vi "HFRR ADV v013 new software.vi"() -> ()   [LabVIEW 2025] (continued)
            n3539 = property class="DigNum (strict)"("Numeric Text.Text Colors:Text Color"="NI Text  2") -> ()  [unwired: 2 in, 2 out]
            n3540 = property class="DigNum (strict)"("Numeric Text.Text Colors:Text Color"="NI Text  2") -> ()  [unwired: 2 in, 2 out]
            n3541 = property class="DigNum (strict)"("Numeric Text.Text Colors:Text Color"="NI Text  2") -> ()  [unwired: 2 in, 2 out]
            n3542 = property on="Coefficient Of Friction" class="XYGraph (strict)"("Plot Area:Colors:FG Color"="GFG  2", "Plot Area:Colors:BG Color"="GBG   2") -> ()  [unwired: 2 in, 2 out]
            n3543 = property on="Humidity ( %RH )" class="XYGraph (strict)"("Plot Area:Colors:FG Color"="GFG  2", "Plot Area:Colors:BG Color"="GBG   2") -> ()  [unwired: 2 in, 2 out]
            n3544 = property on="Air Temperature  ( °C )" class="XYGraph (strict)"("Plot Area:Colors:FG Color"="GFG  2", "Plot Area:Colors:BG Color"="GBG   2") -> ()  [unwired: 2 in, 2 out]
            n3545 = property on="Sample Temperature ( °C )" class="XYGraph (strict)"("Plot Area:Colors:FG Color"="GFG  2", "Plot Area:Colors:BG Color"="GBG   2") -> ()  [unwired: 2 in, 2 out]
            n3546 = property class="DigNum (strict)"("Numeric Text.Text Colors:BG Color"="NI BG 2") -> ()  [unwired: 2 in, 2 out]
            n3547 = property class="DigNum (strict)"("Numeric Text.Text Colors:BG Color"="NI BG 2") -> ()  [unwired: 2 in, 2 out]
            n3548 = property class="DigNum (strict)"("Numeric Text.Text Colors:BG Color"="NI BG 2") -> ()  [unwired: 2 in, 2 out]
            n3549 = property class="DigNum (strict)"("Numeric Text.Text Colors:BG Color"="NI BG 2") -> ()  [unwired: 2 in, 2 out]
            n3550 = property class="DigNum (strict)"("Numeric Text.Text Colors:BG Color"="NI BG 2") -> ()  [unwired: 2 in, 2 out]
            n3551 = property class="DigNum (strict)"("Numeric Text.Text Colors:BG Color"="NI BG 2") -> ()  [unwired: 2 in, 2 out]
            n3552 = property class="DigNum (strict)"("Numeric Text.Text Colors:BG Color"="NI BG 2") -> ()  [unwired: 2 in, 2 out]
            n3553 = property class="DigNum (strict)"("Numeric Text.Text Colors:BG Color"="NI BG 2") -> ()  [unwired: 2 in, 2 out]
            n3554 = property class="DigNum (strict)"("Numeric Text.Text Colors:BG Color"="NI BG 2") -> ()  [unwired: 2 in, 2 out]
            n3555 = property class="DigNum (strict)"("Numeric Text.Text Colors:BG Color"="NI BG 2") -> ()  [unwired: 2 in, 2 out]
            n3556 = property class="DigNum (strict)"("Numeric Text.Text Colors:BG Color"="NI BG 2") -> ()  [unwired: 2 in, 2 out]
            n3557 = property class="DigNum (strict)"("Numeric Text.Text Colors:BG Color"="NI BG 2") -> ()  [unwired: 2 in, 2 out]
            n3558 = property class="DigNum (strict)"("Numeric Text.Text Colors:BG Color"="NI BG 2") -> ()  [unwired: 2 in, 2 out]
            n3559 = property class="DigNum (strict)"("Numeric Text.Text Colors:BG Color"="NI BG 2") -> ()  [unwired: 2 in, 2 out]
            n3560 = property class="DigNum (strict)"("Numeric Text.Text Colors:BG Color"="NI BG 2") -> ()  [unwired: 2 in, 2 out]
            n3561 = property class="Bool"("Colors [4]"="Boolean BC T & BG") -> ()  [unwired: 2 in, 2 out]
            n3562 = property on="Save & Continue" class="Bool (strict)"("Colors [4]"="Boolean BC T & BG") -> ()  [unwired: 2 in, 2 out]
            n3563 = property on="Heater Button" class="Bool (strict)"("Colors [4]"="Boolean BC T & BG") -> ()  [unwired: 2 in, 2 out]
            n3564 = property class="Bool"("Colors [4]"="Boolean BC T & BG") -> ()  [unwired: 2 in, 2 out]
            n3565 = property on="Humidity" class="Bool (strict)"("Colors [4]"="Boolean BC T & BG") -> ()  [unwired: 2 in, 2 out]
            n3566 = property class="Bool (strict)"("Colors [4]"="Boolean BC T & BG") -> ()  [unwired: 2 in, 2 out]
            n3567 = property on="RUN" class="Bool (strict)"("Colors [4]"="Boolean BC T & BG") -> ()  [unwired: 2 in, 2 out]
            n3568 = property on="trip1 8" class="Bool (strict)"("Colors [4]"="Boolean BC T & BG") -> ()  [unwired: 2 in, 2 out]
            n3569 = property class="Bool"("Colors [4]"="Boolean BC T & BG") -> ()  [unwired: 2 in, 2 out]
            n3570 = property class="Bool (strict)"("Colors [4]"="Boolean BC T & BG") -> ()  [unwired: 2 in, 2 out]
            n3571 = property on="OPEN 1" class="Bool (strict)"("Colors [4]"="Boolean BC T & BG 2") -> ()  [unwired: 2 in, 2 out]
            n3572 = property on="OPEN 2" class="Bool (strict)"("Colors [4]"="Boolean BC T & BG 2") -> ()  [unwired: 2 in, 2 out]
            n3573 = property on="OPEN 3" class="Bool (strict)"("Colors [4]"="Boolean BC T & BG 2") -> ()  [unwired: 2 in, 2 out]
            n3574 = property on="OPEN 4" class="Bool (strict)"("Colors [4]"="Boolean BC T & BG 2") -> ()  [unwired: 2 in, 2 out]
            n3575 = property on="OPEN" class="Bool (strict)"("Colors [4]"="Boolean BC T & BG 2") -> ()  [unwired: 2 in, 2 out]
            n3576 = property on="rstv2" class="Bool"("Colors [4]"="Boolean BC T & BG 2") -> ()  [unwired: 2 in, 2 out]
            n3577 = property on="RST CP" class="Bool"("Colors [4]"="Boolean BC T & BG 2") -> ()  [unwired: 2 in, 2 out]
            n3578 = property on="RSTV1 3" class="Bool"("Colors [4]"="Boolean BC T & BG 2") -> ()  [unwired: 2 in, 2 out]
            n3579 = property on="RSTV1 2" class="Bool"("Colors [4]"="Boolean BC T & BG 2") -> ()  [unwired: 2 in, 2 out]
          }
          frame #1 {
          }
        }
        n3580 = local read "Quit"() -> (w4456:bool)
      }
    }
    frame Enabled {
    }
  }
  n3581 = while {
    shift-right: [w4474] -> _
    shift-left: _ -> [w4475]
    shift-right: [w4472] -> _
    shift-left: T18 {"Read Heave and Surge"="", "Bytes at Heave Port"=0.0, "Heave and Surge COM Port:"="COM9", "Com Port 2"="COM7", "Residual Due"="", "Heave COM Status 2"=TRUE, "Heave COM Status"=TRUE, "Port 2"=TRUE, "Sway PPR"=6400.0, "Surge PPR"=6400.0, "Heave PPR"=6400.0, "Sway Pitch"=2.0, "Surge Pitch"=3.0, "Heave Pitch"=4.0, "Sway Pulses/mm"=320.0, "Surge Pulses/mm"=1600.0, "Heave Pulses/mm"=1600.0, "inner loop"=0.0, "Read Heave and Surge 2"="", "String 36"="", "Write S"=FALSE, "WriteCC1"=[""], "Heave COM Loop"=0, "LastCom"="", "EXIT"=FALSE, "Error Heave"={"status"=TRUE, "code"=-1073807343, "source"=""}} -> [w4471]
    shift-right: [w4469] -> _
    shift-left: enum16{"init", "MAIN", "Panel Close"}."init" -> [w4470]
    stop <- w4473 stop-if-true
    n3582 = case shown="\"MAIN\"" w4470 {
      tunnel: w4475 -> [w4489 w4504 w4565 w4567]
      tunnel: [w4483 w4513 w4565 w4567] -> w4474
      tunnel: [_ _ TRUE _] -> w4473
      tunnel: [w4479 w4510 w4563 w4566] -> w4472
      tunnel: w4471 -> [w4486 w4503 w4563 w4566]
      tunnel: [enum16{"init", "MAIN", "Panel Close"}."MAIN" w4497 _ _] -> w4469
      frame "init" {
        n3583 = Bundle By Name(cluster=w4486, "Heave and Surge COM Port:"="C3 :") -> (w4485:T18)
        n3584 = call "Instrument fgv.vi"("Enum"=T30."INIT", "error in (no error) 2"=w4489, "INPUT"=w4485) -> ("error"=w4487:errorcluster, "output"=w4482:T18)  [unwired: 6 in, 1 out]
        n3585 = case shown="Error" w4487 {
          selector: w4487 -> [w4491 _]
          tunnel: [w4491 w4495] -> w4483
          tunnel: w4482 -> [w4490 w4493]
          tunnel: [w4490 w4492] -> w4480
          frame No Error {
          }
          frame Error {
            n3586 = call "Instrument fgv.vi"("Enum"=T30."ERROR INIT", "INPUT"=w4493) -> ("error"=w4496:errorcluster, "output"=w4492:T18)  [unwired: 7 in, 1 out]
            n3587 = call <vilib>:"Clear Errors.vi"("error in (no error)"=w4496) -> ("error out"=w4495:errorcluster)  [unwired: 5 in, 1 out]
          }
        }
        n3588 = local read "LastCom"() -> (w4478:string)
        n3589 = Unbundle By Name(w4480) -> ("Heave COM Status 2"=→"COM Status" →"Instrument Status":bool, "Error Heave"=→"Error":errorcluster)  [unwired: 1 out]
        n3590 = Bundle By Name(cluster=w4480, "LastCom"=w4478) -> (w4479:T18)
      }
      frame "MAIN" {
        n3591 = Unbundle By Name(w4503) -> ("Com Port 2"=w4515:refnum<visa-resource-name>)
        n3592 = local write "Com Port 4"(w4515) -> ()
        n3593 = local read "C3 :"() -> (w4501:refnum<visa-resource-name>)
        n3594 = Bundle By Name(cluster=w4503, "Heave and Surge COM Port:"=w4501) -> (w4502:T18)
        n3595 = Equal?(x=w4515, y=w4501) -> (x = y?=w4514:bool)
        n3596 = case shown="True" w4514 {
          tunnel: [w4519 w4536] -> w4513
          tunnel: w4504 -> [w4520 w4542]
          tunnel: w4502 -> [w4518 w4540]
          tunnel: [w4517 w4535] -> w4510
          frame False {
            n3597 = call <vilib>:"Clear Errors.vi"("error in (no error)"=w4520) -> ("error out"=w4516:errorcluster)  [unwired: 5 in, 1 out]
            n3598 = call "Instrument fgv.vi"("Enum"=T30."ERROR INIT", "error in (no error) 2"=w4516, "INPUT"=w4518) -> ("error"=w4522:errorcluster, "output"=w4517:T18)  [unwired: 6 in, 1 out]
            n3599 = call <vilib>:"Clear Errors.vi"("error in (no error)"=w4522) -> ("error out"=w4519:errorcluster)  [unwired: 5 in, 1 out]
          }
          frame True {
            n3600 = call "Instrument fgv.vi"("Enum"=T30."READ", "error in (no error) 2"=w4542, "INPUT"=w4540) -> ("error"=w4541:errorcluster, "output"=w4532:T18)  [unwired: 6 in, 1 out]
            n3601 = Bundle By Name(cluster=w4532, "String 36"="String 11") -> (w4531:T18)
            n3602 = case shown="True" "Write S" {
              selector: "Write S" -> [_ w4562]
              tunnel: w4541 -> [w4555 w4561]
              tunnel: [w4555 w4560] -> w4528
              tunnel: w4531 -> [w4554 w4557]
              tunnel: [w4554 w4556] -> w4527
              frame False {
              }
              frame True {
                n3603 = Not(x=w4562) -> (.not. x?=w4558:bool)
                n3604 = local write "Write S"(w4558) -> ()
                n3605 = call "Instrument fgv.vi"("Enum"=T30."MANUAL WRITE", "error in (no error) 2"=w4561, "INPUT"=w4557) -> ("error"=w4560:errorcluster, "output"=w4556:T18)  [unwired: 6 in, 1 out]
              }
            }
            n3606 = Array Size(array="WriteHumidity") -> (size(s)=w4525:i32)
            n3607 = Greater Than 0?(x=w4525) -> (x > 0?=w4523:bool)
            n3608 = call "Instrument fgv.vi"("Enum"=T30."WRITE", "error in (no error) 2"=w4528, "WriteCC1"="WriteHumidity", "INPUT"=w4527) -> ("error"=w4538:errorcluster, "WriteCC1 2"=w4526:string[], "output"=w4537:T18)  [unwired: 5 in]
            n3609 = case shown="True" w4523 {
              tunnel: w4526 -> [_ w4544]
              frame False {
              }
              frame True {
                n3610 = local write "WriteHumidity"(w4544) -> ()
              }
            }
            n3611 = case shown="Error" w4538 {
              selector: w4538 -> [w4545 w4548]
              tunnel: w4537 -> [w4546 w4553]
              tunnel: [w4546 w4552] -> w4535
              tunnel: [w4545 w4550] -> w4536
              frame No Error {
              }
              frame Error {
                n3612 = call <vilib>:"Clear Errors.vi"("error in (no error)"=w4548) -> ("error out"=w4547:errorcluster)  [unwired: 5 in, 1 out]
                n3613 = call "Instrument fgv.vi"("Enum"=T30."ERROR INIT", "error in (no error) 2"=w4547, "INPUT"=w4553) -> ("error"=w4551:errorcluster, "output"=w4552:T18)  [unwired: 6 in, 1 out]
                n3614 = call <vilib>:"Clear Errors.vi"("error in (no error)"=w4551) -> ("error out"=w4550:errorcluster)  [unwired: 5 in, 1 out]
              }
            }
            n3615 = Unbundle By Name(w4535) -> ("LastCom"=→"LastCom":string, "Read Heave and Surge"=→"Read Humidity":string)
          }
        }
        n3616 = Unbundle By Name(w4510) -> ("Heave COM Status 2"=w4512:bool, "Heave COM Status"=w4511:bool, "Error Heave"=w4508:errorcluster, "Bytes at Heave Port"=→"Bytes at Humidity Port":dbl)
        n3617 = Unbundle By Name(w4508) -> ("status"=→"Humidity Port":bool)
        n3618 = Not(x=w4511) -> (.not. x?=w4505:bool)
        n3619 = local write "Error"(w4508) -> ()
        n3620 = Not(x=w4512) -> (.not. x?=w4506:bool)
        n3621 = local write "Instrument Status"(w4505) -> ()
        n3622 = local write "COM Status"(w4506) -> ()
        n3623 = local read "Quit"() -> (w4498:bool)
        n3624 = Select(t=enum16{"init", "MAIN", "Panel Close"}."Panel Close", s=w4498, f=enum16{"init", "MAIN", "Panel Close"}."MAIN") -> (s? t:f=w4497:enum16{"init", "MAIN", "Panel Close"})
      }
      frame "Panel Close" {
      }
      frame Default {
      }
    }
  }
  n3625 = while {
    stop <- w4593 stop-if-true
    n3626 = local read "Read Humidity"() -> (w4574:string)
    n3627 = call <vilib>:"High Resolution Polling Wait.vi"("seconds to wait"=0.1) -> ()  [unwired: 10 in, 1 out]
    n3628 = Spreadsheet String To Array(delimiter (Tab)=",", format string="", spreadsheet string=w4574, array type (2D Dbl)=string[] []) -> (array=w4588:string[])
    n3629 = for {
      tunnel: w4588 -> [w4598] mode=indexing
      tunnel: string[] ["STATE;", "SET;", "RH;", "T;", "AMB_RH;", "AMB_T;", "PUMP;", "FAN_IN;", "FAN_OUT;", "DEHUM;", "CURRENT;", "STALL;"] -> [w4597] mode=indexing
      tunnel: [w4596] -> w4587 mode=indexing
      n3630 = Match Pattern(string=w4598, regular expression=w4597) -> (after substring=w4596:string)  [unwired: 1 in, 3 out]
    }
    n3631 = Index Array(array=w4587) -> (element #1=→"STATE :":string, element #2=→"SET :":string, element #3=w4576:string, element #4=→"T :":string, element #5=w4573:string, element #6=→"AMB_T :":string, element #7=→"PUMP :":string, element #8=→"FAN_IN :":string, element #9=→"FAN_OUT :":string, element #10=→"DEHUM :":string, element #11=→"CURRENT :":string, element #12=→"STALL :":string)  [unwired: 12 in]
    "RH :" <- w4576
    "AMB_RH :" <- w4573
    n3632 = Fract/Exp String To Number(string=w4576) -> (number=w4568:dbl)  [unwired: 3 in, 1 out]
    n3633 = Fract/Exp String To Number(string=w4573) -> (number=w4572:dbl)  [unwired: 3 in, 1 out]
    n3634 = local write "Ambient Humidity :"(w4572) -> ()
    n3635 = Equal?(x=w4568, y=0.0) -> (x = y?=w4570:bool)
    n3636 = case shown="True" w4570 {
      tunnel: [w4594 w4595] -> w4569
      tunnel: w4568 -> [w4594 _]
      frame False {
        (unwired) 0.0
        "Humidity temp" <- w4594
      }
      frame True {
        n3637 = local read "Humidity temp"() -> (w4595:dbl)
      }
    }
    "RH Numeric:" <- w4569
    n3638 = local read "Quit"() -> (w4593:bool)
  }
  n3639 = disable-structure shown="Disabled" {
    frame Disabled {
      n3640 = while {
        tunnel: [w4832] -> _
        i -> [w4832]
        stop <- w4829 stop-if-true
        n3641 = local read "powstat"() -> (w4830:bool)
        n3642 = case shown="True" w4830 {
          frame False {
          }
          frame True {
            n3643 = local read "RUN"() -> (w4833:bool)
            n3644 = case shown="True" w4833 {
              frame False {
                w4863 = 65.0 ("y")
                n3645 = local read "Set Hz"() -> (w4891:dbl)
                n3646 = local read "NORMAL LOAD"() -> (w4892:dbl)
                n3647 = Multiply(x=w4891, y=60.0) -> (x*y=w4898:dbl)
                n3648 = Multiply(x=1.2 ("y"), y=0.949) -> (x*y=w4867:dbl)
                n3649 = Multiply(x=1.2 ("y"), y=0.8166) -> (x*y=w4871:dbl)
                n3650 = Multiply(x=1.2 ("y"), y=0.851) -> (x*y=w4866:dbl)
                n3651 = local read "FF 2"() -> (w4890:dbl)
                n3652 = Absolute Value(x=w4898) -> (abs(x)=w4896:dbl)
                n3653 = case shown="13.." w4890 {
                  tunnel: [1 2 3] -> w4888
                  frame 0..10, Default {
                    # "Normal"
                  }
                  frame 11, 12 {
                  }
                  frame 13.. {
                  }
                }
                "FF STATE" <- w4888
                n3654 = local read "TEMP"() -> (w4851:dbl)
                n3655 = local read item#-1() -> (w4865)
                n3656 = Less?(x=w4865, y=w4871) -> (x < y?=w4868:bool)
                n3657 = In Range and Coerce(upper limit=w4867, x=w4865, lower limit=w4866) -> (In Range?=w4869:bool)  [unwired: 1 out]
                n3658 = case shown="3601.." w4896 {
                  tunnel: [1 2 3] -> w4894
                  frame 0..3000, Default {
                    # "Normal"
                  }
                  frame 3001..3600 {
                  }
                  frame 3601.. {
                  }
                }
                n3659 = case shown="11.." w4892 {
                  tunnel: [1 3] -> w4893
                  frame 1..10, Default {
                  }
                  frame 11.. {
                  }
                }
                "NL STATE" <- w4893
                n3660 = Multiply(x=1.2 ("y"), y=0.95) -> (x*y=w4881:dbl)
                n3661 = Multiply(x=w4863, y=0.954) -> (x*y=w4855:dbl)
                n3662 = Or(x=w4868, y=w4869) -> (x .or. y?=w4870:bool)
                n3663 = Greater Or Equal?(x=w4865, y=w4881) -> (x >= y?=w4878:bool)
                n3664 = Multiply(x=w4863, y=0.99) -> (x*y=w4852:dbl)
                n3665 = Greater Or Equal?(x=w4851, y=w4852) -> (x >= y?=w4857:bool)
                n3666 = Greater Or Equal?(x=w4851, y=w4855) -> (x >= y?=w4854:bool)
                n3667 = case shown="0, 1, Default" w4865 {
                  tunnel: [1 3] -> w4882
                  frame 0, 1, Default {
                  }
                  frame 2.. {
                  }
                }
                n3668 = case shown="True" w4878 {
                  tunnel: [1 3] -> w4883
                  frame False {
                  }
                  frame True {
                  }
                }
                n3669 = case shown="True" w4870 {
                  tunnel: [1 2] -> w4884
                  frame False {
                  }
                  frame True {
                  }
                }
                n3670 = case shown="..0" w4851 {
                  tunnel: [2 3 3 1] -> w4858
                  frame 61, 62 {
                  }
                  frame 63.. {
                  }
                  frame ..0 {
                  }
                  frame 10..60, Default {
                  }
                }
                n3671 = case shown="True" w4857 {
                  tunnel: [1 3] -> w4859
                  frame False {
                  }
                  frame True {
                  }
                }
                n3672 = Number To Decimal String(number=w4894) -> (decimal integer string=w4895:string)  [unwired: 1 in]
                n3673 = case shown="True" w4854 {
                  tunnel: [1 2] -> w4860
                  frame False {
                  }
                  frame True {
                  }
                }
                n3674 = Number To Decimal String(number=1) -> (decimal integer string=→"Air temp":string)  [unwired: 1 in]
                n3675 = Number To Decimal String(number=w4888) -> (decimal integer string=→"ff_st":string)  [unwired: 1 in]
                n3676 = local write "sp_st"(w4895) -> ()
                n3677 = Number To Decimal String(number=w4893) -> (decimal integer string=→"nl_st":string)  [unwired: 1 in]
                n3678 = Build Array(w4858, w4859, w4860) -> (w4861:i32[])
                n3679 = Build Array(w4882, w4883, w4884) -> (w4885:i32[])
                n3680 = Array Max & Min(array=w4861) -> (max value=w4862:i32)  [unwired: 3 out]
                n3681 = Array Max & Min(array=w4885) -> (max value=w4886:i32)  [unwired: 3 out]
                n3682 = Number To Decimal String(number=w4862) -> (decimal integer string=w4850:string)  [unwired: 1 in]
                n3683 = Number To Decimal String(number=w4886) -> (decimal integer string=→"Stroke Ln 2":string)  [unwired: 1 in]
                n3684 = local write "temp_st"(w4850) -> ()
              }
              frame True {
                w4948 = 65.0 ("y")
                # "Healthy -1\nWarning -2\nError -3"
                n3685 = local read "TEMP"() -> (w4959:dbl)
                n3686 = local read "NORMAL LOAD"() -> (w4963:dbl)
                n3687 = local read "Set Hz"() -> (w4961:dbl)
                n3688 = Multiply(x=1.2 ("y"), y=0.949) -> (x*y=w4943:dbl)
                n3689 = Multiply(x=1.2 ("y"), y=0.8166) -> (x*y=w4939:dbl)
                n3690 = Multiply(x=1.2 ("y"), y=0.851) -> (x*y=w4944:dbl)
                n3691 = Multiply(x=w4948, y=0.954) -> (x*y=w4955:dbl)
                n3692 = Multiply(x=w4948, y=0.99) -> (x*y=w4958:dbl)
                n3693 = Greater Or Equal?(x=w4959, y=w4958) -> (x >= y?=w4953:bool)
                n3694 = Multiply(x=w4961, y=60.0) -> (x*y=w4967:dbl)
                n3695 = Greater Or Equal?(x=w4959, y=w4955) -> (x >= y?=w4956:bool)
                n3696 = local read "FF 2"() -> (w4962:dbl)
                n3697 = local read item#-1() -> (w4945)
                n3698 = Less?(x=w4945, y=w4939) -> (x < y?=w4942:bool)
                n3699 = In Range and Coerce(upper limit=w4943, x=w4945, lower limit=w4944) -> (In Range?=w4941:bool)  [unwired: 1 out]
                n3700 = Absolute Value(x=w4967) -> (abs(x)=w4965:dbl)
                n3701 = case shown="63.." w4959 {
                  tunnel: [2 3 3 1] -> w4952
                  frame 61, 62 {
                  }
                  frame 63.. {
                  }
                  frame ..0 {
                  }
                  frame 10..60, Default {
                  }
                }
                n3702 = case shown="True" w4953 {
                  tunnel: [1 3] -> w4951
                  frame False {
                  }
                  frame True {
                  }
                }
                n3703 = case shown="True" w4956 {
                  tunnel: [1 2] -> w4950
                  frame False {
                  }
                  frame True {
                  }
                }
                n3704 = Multiply(x=1.2 ("y"), y=0.95) -> (x*y=w4929:dbl)
                n3705 = case shown="1..10, Default" w4963 {
                  tunnel: [1 3] -> w4970
                  frame 1..10, Default {
                  }
                  frame 11.. {
                  }
                }
                n3706 = case shown="0..10, Default" w4962 {
                  tunnel: [1 2 3] -> w4969
                  frame 0..10, Default {
                  }
                  frame 11, 12 {
                  }
                  frame 13.. {
                  }
                }
                n3707 = case shown="3601.." w4965 {
                  tunnel: [1 2 3] -> w4964
                  frame 0..3000, Default {
                    # "Normal"
                  }
                  frame 3001..3600 {
                  }
                  frame 3601.. {
                  }
                }
                n3708 = Or(x=w4942, y=w4941) -> (x .or. y?=w4940:bool)
                n3709 = Greater Or Equal?(x=w4945, y=w4929) -> (x >= y?=w4932:bool)
                n3710 = case shown="0, 1, Default" w4945 {
                  tunnel: [1 3] -> w4928
                  frame 0, 1, Default {
                  }
                  frame 2.. {
                  }
                }
                n3711 = case shown="True" w4932 {
                  tunnel: [1 3] -> w4927
                  frame False {
                  }
                  frame True {
                  }
                }
                n3712 = case shown="True" w4940 {
                  tunnel: [1 2] -> w4926
                  frame False {
                  }
                  frame True {
                  }
                }
                n3713 = Build Array(w4952, w4951, w4950) -> (w4949:i32[])
                n3714 = Number To Decimal String(number=w4964) -> (decimal integer string=→"sp_st":string)  [unwired: 1 in]
                n3715 = Array Max & Min(array=w4949) -> (max value=w4946:i32)  [unwired: 3 out]
                "TEMP STATE" <- w4946
                n3716 = Number To Decimal String(number=w4970) -> (decimal integer string=w4973:string)  [unwired: 1 in]
                n3717 = Number To Decimal String(number=w4969) -> (decimal integer string=w4971:string)  [unwired: 1 in]
                n3718 = Number To Decimal String(number=w4946) -> (decimal integer string=→"temp_st":string)  [unwired: 1 in]
                n3719 = Build Array(w4928, w4927, w4926) -> (w4925:i32[])
                n3720 = local write "nl_st"(w4973) -> ()
                n3721 = local write "ff_st"(w4971) -> ()
                n3722 = Number To Decimal String(number=1) -> (decimal integer string=w4968:string)  [unwired: 1 in]
                n3723 = Array Max & Min(array=w4925) -> (max value=w4924:i32)  [unwired: 3 out]
                n3724 = local write "Air temp"(w4968) -> ()
                n3725 = Number To Decimal String(number=w4924) -> (decimal integer string=w4923:string)  [unwired: 1 in]
                n3726 = local write "Stroke Ln 2"(w4923) -> ()
              }
            }
            n3727 = local read "Stroke Ln 2"() -> (w4835:string)
            n3728 = local read "nl_st"() -> (w4841:string)
            n3729 = local read "ff_st"() -> (w4838:string)
            n3730 = local read "sp_st"() -> (w4839:string)
            n3731 = local read "temp_st"() -> (w4840:string)
            n3732 = local read "Air temp"() -> (w4834:string)
            n3733 = Replace Array Subset(array="in", new element #1=w4841, index #1=1 ("index"), new element #2=w4838, index #2=2 ("index"), new element #3=w4840, index #3=3 ("index"), new element #4=w4839, index #4=4 ("index"), new element #5=w4835, index #5=5 ("index"), new element #6=w4834, index #6=6 ("index"), new element #7="Sensor State" ("new element/subarray"), index #7=0 ("index")) -> (→"out":string[])
          }
        }
        n3734 = Wait (ms)(milliseconds to wait=u32 10) -> ()  [unwired: 1 out]
        n3735 = local read "Quit"() -> (w4829:bool)
      }
      n3736 = while {
        stop <- w4804 stop-if-true
        n3737 = local read "run replace"() -> (w4806:bool)
        n3738 = Wait (ms)(milliseconds to wait=u32 100) -> ()  [unwired: 1 out]
        n3739 = Equal?(x="FLAG 2", y=0.0) -> (x = y?=w4807:bool)
        n3740 = case shown="True" w4807 {
          frame False {
          }
          frame True {
            n3741 = local write "FLAG 2"(100.0 ("FLAG 2")) -> ()
            n3742 = call <vilib>:"Read Characters From File.vi"("file path (dialog if empty)"=path "C:/LAB-IQ-NXT/WO 2449 TT.sig", "convert eol? (no:F)"=FALSE ("append to file? (new file:F)")) -> ("character string"=w4810:string)  [unwired: 4 in, 3 out]
            n3743 = call <vilib>:"Read Characters From File.vi"("file path (dialog if empty)"=path "C:/LAB-IQ-NXT/WO 2449 TRH.sig", "convert eol? (no:F)"=FALSE ("append to file? (new file:F)")) -> ("character string"=w4811:string)  [unwired: 4 in, 3 out]
            n3744 = Decimal String To Number(string=w4810) -> (number=w4812:i32)  [unwired: 2 in, 1 out]
            n3745 = local write "Total No. of Tests"(w4812) -> ()
            n3746 = Decimal String To Number(string=w4811) -> (number=w4815:i32)  [unwired: 2 in, 1 out]
            n3747 = local write "SEN.RUN HRS"(w4815) -> ()
          }
        }
        n3748 = case shown="True" w4806 {
          frame False {
          }
          frame True {
            n3749 = Equal?(x="FLAG 4", y=0.0) -> (x = y?=w4819:bool)
            n3750 = case shown="False" w4819 {
              frame False {
                n3751 = Get Date/Time In Seconds() -> (seconds since 1Jan1904=w4825:timestamp)
                n3752 = local read "START 3"() -> (w4823:dbl)
                n3753 = To Double Precision Float(number=w4825) -> (double precision float=w4824:dbl)
                n3754 = Subtract(x=w4824, y=w4823) -> (x-y=→"SENSOR TIME":dbl)
              }
              frame True {
                n3755 = Get Date/Time In Seconds() -> (seconds since 1Jan1904=w4827:timestamp)
                n3756 = local write "FLAG 4"(100.0 ("FLAG")) -> ()
                n3757 = To Double Precision Float(number=w4827) -> (double precision float=→"START 3":dbl)
              }
            }
          }
        }
        n3758 = local read "Quit"() -> (w4804:bool)
      }
      n3759 = while {
        shift-right: [w4604] -> _
        shift-left: _ -> [w4605]
        tunnel: [w4600] -> _
        i -> [w4600]
        stop <- w4599 stop-if-true
        n3760 = Wait (ms)(milliseconds to wait=u32 50 ("Refresh Rate (ms)")) -> ()  [unwired: 1 out]
        n3761 = local read "Json End Flg"() -> (w4601:bool)
        n3762 = Not(x="Upld AR 2") -> ()  [unwired: 1 out]
        n3763 = local read "Upld AR 2"() -> (w4602:bool)
        n3764 = call "Elapsed Time9"("Time Target (s)"="Sen.Upload Rate (s)", "Reset"=FALSE, "Auto Reset"=TRUE) -> ("Time has Elapsed"=w4611:bool)  [unwired: 9 in, 7 out]
        n3765 = Or(x=w4611, y=w4601) -> (x .or. y?=w4607:bool)
        n3766 = case shown="True" w4607 {
          frame False {
          }
          frame True {
            w4703 = "\"SensorName\":\"" ("string")
            w4673 = " \"},{"
            w4698 = "\",\"SensorState\":\""
            w4700 = "\",\"SensorModelNumber\":\"" ("string")
            w4699 = "\",\"SensorRuntimeHours\":\"" ("string")
            n3767 = local read "model num"() -> (w4697:string[])
            n3768 = local read "Sensor name"() -> (w4716:string[])
            n3769 = local read "run"() -> (w4687:string[])
            n3770 = local read "SENSOR TIME"() -> (w4643:dbl)
            n3771 = local read "out"() -> (w4636:string[])
            n3772 = local read "Total No. of Tests"() -> (w4641:dbl)
            n3773 = Select(t=60.0, s="Run test 3", f=3600.0) -> (s? t:f=w4651:dbl)
            n3774 = Index Array(array=w4697, index #1=1 ("index")) -> (element #1=w4696:string, element #2=w4695:string, element #3=w4694:string, element #4=w4693:string, element #5=w4692:string, element #6=w4691:string)  [unwired: 5 in]
            n3775 = Index Array(array=w4687, index #1=1 ("index")) -> (element #1=w4686:string, element #2=w4685:string, element #3=w4684:string, element #4=w4683:string, element #5=w4682:string, element #6=w4681:string)  [unwired: 5 in]
            n3776 = Index Array(array=w4716, index #1=1 ("index")) -> (element #1=w4715:string, element #2=w4714:string, element #3=w4713:string, element #4=w4712:string, element #5=w4702:string, element #6=w4701:string)  [unwired: 5 in]
            n3777 = Index Array(array=w4636, index #1=1 ("index")) -> (element #1=w4668:string, element #2=w4667:string, element #3=w4666:string, element #4=w4665:string, element #5=w4664:string, element #6=w4663:string)  [unwired: 5 in]
            n3778 = local read "SEN.RUN HRS"() -> (w4639:dbl)
            n3779 = Divide(x=w4643, y=w4651) -> (x/y=w4650:dbl)
            n3780 = Increment(x=w4650) -> (x+1=w4646:dbl)
            n3781 = Number To Decimal String(number=w4646) -> (decimal integer string=→"run hrs":string)  [unwired: 1 in]
            n3782 = Divide(x=w4639, y=3600.0 ("f")) -> (x/y=w4634:dbl)
            n3783 = Round To Nearest(number=w4634) -> (nearest integer value=w4632:dbl)
            n3784 = Number To Decimal String(number=w4632) -> (decimal integer string=w4633:string)  [unwired: 1 in]
            n3785 = Number To Decimal String(number=w4641) -> (decimal integer string=w4642:string)  [unwired: 1 in]
            n3786 = local read "Model No"() -> (w4647:string)
            n3787 = local read "UUID"() -> (w4742:string)
            n3788 = local read "Serial No"() -> (w4746:string)
            n3789 = local read "Secret Key"() -> (w4747:string)
            n3790 = Concatenate Strings("\",\"MachineSerialNumber\":\"" ("string"), w4746) -> (w4750:string)
            n3791 = Concatenate Strings("\",\"ModelNumber\":\"" ("string"), w4647) -> (w4648:string)
            n3792 = Concatenate Strings("\",\"MachineRuntimeHours\":\"" ("string"), w4633) -> (w4751:string)
            n3793 = Concatenate Strings("\",\"MachineRuntimeCycles\":\"", w4642) -> (w4744:string)
            n3794 = Concatenate Strings(w4700, w4696) -> (w4730:string)
            n3795 = Concatenate Strings(w4699, w4686) -> (w4731:string)
            n3796 = Concatenate Strings(w4698, w4668) -> (w4729:string)
            n3797 = Concatenate Strings(w4750, w4648, w4751, w4744) -> (w4753:string)
            n3798 = Concatenate Strings(w4700, w4695) -> (w4727:string)
            n3799 = Concatenate Strings(w4699, w4685) -> (w4726:string)
            n3800 = Concatenate Strings(w4698, w4667) -> (w4728:string)
            n3801 = Concatenate Strings(w4700, w4694) -> (w4722:string)
            n3802 = Concatenate Strings(w4699, w4684) -> (w4723:string)
            n3803 = Concatenate Strings(w4698, w4666) -> (w4721:string)
            n3804 = Concatenate Strings(w4700, w4693) -> (w4719:string)
            n3805 = Concatenate Strings(w4699, w4683) -> (w4718:string)
            n3806 = Concatenate Strings(w4698, w4665) -> (w4720:string)
            n3807 = Concatenate Strings(w4730, w4731, w4729) -> (w4732:string)
            n3808 = Concatenate Strings(w4700, w4692) -> (w4709:string)
            n3809 = Concatenate Strings(w4699, w4682) -> (w4710:string)
            n3810 = Concatenate Strings(w4700, w4691) -> (w4706:string)
            n3811 = Concatenate Strings(w4699, w4681) -> (w4705:string)
            n3812 = Concatenate Strings(w4698, w4664) -> (w4708:string)
            n3813 = Concatenate Strings(w4698, w4663) -> (w4707:string)
            n3814 = Concatenate Strings("{\"SecretKey\":\"", w4747, w4753, "\",\"UUID\" : \"", w4742, "\",\"SensorInformation\":", "[{" ("string")) -> (w4680:string)
            n3815 = Concatenate Strings(w4727, w4726, w4728) -> (w4725:string)
            n3816 = Concatenate Strings(w4722, w4723, w4721) -> (w4724:string)
            n3817 = Concatenate Strings(w4719, w4718, w4720) -> (w4717:string)
            n3818 = Concatenate Strings(w4709, w4710, w4708) -> (w4711:string)
            n3819 = Concatenate Strings(w4706, w4705, w4707) -> (w4704:string)
            n3820 = Concatenate Strings(w4703, w4715, w4732, w4673) -> (w4679:string)
            n3821 = Concatenate Strings(w4703, w4714, w4725, w4673) -> (w4678:string)
            n3822 = Concatenate Strings(w4703, w4713, w4724, w4673) -> (w4677:string)
            n3823 = Concatenate Strings(w4703, w4712, w4717, w4673) -> (w4676:string)
            n3824 = Concatenate Strings(w4703, w4702, w4711, w4673) -> (w4675:string)
            n3825 = Concatenate Strings(w4703, w4701, w4704, "\"}" ("string")) -> (w4674:string)
            n3826 = Concatenate Strings(w4680, w4679, w4678, w4677, w4676, w4675, w4674, "]}" ("string")) -> (w4671:string)
            n3827 = local read "SEN.RUN HRS"() -> (w4638:dbl)
            n3828 = disable-structure shown="Disabled" {
              frame Disabled {
                n3829 = local read "state"() -> (w4757:string[])
                n3830 = Delete From Array(array=w4757, index=0) -> (array with subset deleted=w4755:string[])  [unwired: 1 in, 1 out]
                n3831 = for {
                  N: 6 -> [_]
                  tunnel: w4755 -> [w4768] mode=indexing
                  tunnel: [w4767] -> w4754 mode=indexing
                  n3832 = Equal?(x=w4768, y="Warning") -> (x = y?=w4764:bool)
                  n3833 = Equal?(x=w4768, y="Healthy") -> (x = y?=w4761:bool)
                  n3834 = Select(t="2" ("y"), s=w4764, f="3" ("y")) -> (s? t:f=w4759:string)
                  n3835 = Select(t="1" ("y"), s=w4761, f=w4759) -> (s? t:f=w4767:string)
                }
                "state1" <- w4754
              }
              frame Enabled {
              }
            }
            n3836 = stacked-sequence {
              tunnel: w4671 -> [w4779 _ _]
              tunnel: [_ _ w4795] -> _
              frame #0 {
                (unwired) FALSE ("convert eol (F)")
                w4781 = enum16{"start", "end", "current"}."start" ("pos mode (0:2)")
                n3837 = local read "Path"() -> (w4775:path)
                n3838 = Path To String(path=w4775) -> (string=w4787:string)
                n3839 = Concatenate Strings(w4787, "\\", "Sensor File Name") -> (w4788:string)
                n3840 = local write "standard output 2"(" ") -> ()
                n3841 = String To Path(string=w4788) -> (path=w4778:path)
                n3842 = call <vilib>:"Open_Create_Replace File.vi"("advisory dialog? (display:T)"=FALSE, "function (open:0)"=T31."create or replace", "file path"=w4778) -> ("error out"=w4791:errorcluster, "refnum"=w4790:refnum<file>)  [unwired: 5 in, 2 out]
                n3843 = Set File Position(refnum=w4790, from (0:start)=w4781, error in=w4791) -> (refnum out=w4771:refnum<file>, error out=w4770:errorcluster)  [unwired: 1 in]
                n3844 = Write to Binary File(file (use dialog)=w4771, data=" ", error in=w4770, 5:FALSE ("prepend array or string size? (T)")) -> (refnum out=w4782:refnum<file>, error out=w4783:errorcluster)  [unwired: 2 in, 1 out]
                n3845 = Set File Position(offset (in bytes) (0)=w4781, refnum=w4782, error in=w4783) -> (refnum out=w4774:refnum<file>, error out=w4773:errorcluster)  [unwired: 1 in]
                n3846 = Write to Binary File(file (use dialog)=w4774, data=w4779, error in=w4773, 5:FALSE ("prepend array or string size? (T)")) -> (error out=w4777:errorcluster)  [unwired: 2 in, 2 out]
                n3847 = flat-sequence {
                  tunnel: w4778 -> [w4793]
                  tunnel: w4777 -> [_]
                  frame #0 {
                    n3848 = call <vilib>:"Read Characters From File.vi"("file path (dialog if empty)"=w4793) -> ("character string"=→"Sensor Health JSON string":string)  [unwired: 5 in, 3 out]
                  }
                }
                "SinglePoint  2" <- w4779
              }
              frame #1 {
              }
              frame #2 {
                (unwired) "\"Stored\": true" ("string")
                n3849 = call <vilib>:"System Exec.vi"("run minimized? (F)"=TRUE, "wait until completion? (T)"=TRUE, "working directory"=path "C:/LAB-IQ-NXT", "command line"="C:\\LAB-IQ-NXT\\JPostH.bat") -> ("standard error"=→"Respose From Server 2":string, "standard output"=w4798:string)  [unwired: 4 in, 2 out]
                "standard output 2" <- w4798
                n3850 = Match Pattern(string=w4798, regular expression="JSONH Check String") -> (match substring=w4796:string, offset past match=w4795:i32)  [unwired: 1 in, 2 out]
                n3851 = Equal?(x=w4796, y="JSONH Check String") -> (x = y?=→"Upload \nConfirmed 2":bool)
              }
            }
            n3852 = Divide(x=w4638, y=3600.0 ("f")) -> (x/y=w4631:dbl)
            n3853 = local read "run time"() -> (w4688:string[])
            n3854 = Round To Nearest(number=w4631) -> (nearest integer value=w4630:dbl)
            n3855 = Number To Decimal String(number=w4630) -> (decimal integer string=w4629:string)  [unwired: 1 in]
            n3856 = Index Array(array="Sensor Information", index (col) #1=0 ("disabled index (col)"), index (col) #2=1 ("index (col)"), index (col) #3=2 ("index (col)"), index (col) #4=3 ("index (col)")) -> (element #1=→"Sensor name":string[], element #2=→"model num":string[], element #3=→"run time":string[], element #4=→"state":string[])  [unwired: 4 in]
            n3857 = Insert Into Array(array=w4688, index=1, new element #1=w4629, new element #2=w4629, new element #3=w4629, new element #4=w4629, new element #5=w4629, new element #6=w4629) -> (w4653:string[])
            "run" <- w4653
            n3858 = local read "out"() -> (w4635:string[])
            n3859 = local read "Sensor Information"() -> (w4655:string[][])
            n3860 = Replace Array Subset(array=w4655, new element #1=w4653, index (col) #1=2 ("disabled index (col)"), new element #2=w4635, index (col) #2=3 ("index (col)")) -> (w4654:string[][])  [unwired: 2 in]
            n3861 = local write "Sensor Information"(w4654) -> ()
          }
        }
        n3862 = case shown="True" w4602 {
          frame False {
          }
          frame True {
            n3863 = Equal?(x="FLAG", y=0.0) -> (x = y?=w4619:bool)
            n3864 = case shown="False" w4619 {
              frame False {
                n3865 = Get Date/Time In Seconds() -> (seconds since 1Jan1904=w4625:timestamp)
                n3866 = local read "START 2"() -> (w4623:dbl)
                n3867 = To Double Precision Float(number=w4625) -> (double precision float=w4624:dbl)
                n3868 = Subtract(x=w4624, y=w4623) -> (x-y=→"SENSOR TIME  2":dbl)
              }
              frame True {
                n3869 = Get Date/Time In Seconds() -> (seconds since 1Jan1904=w4627:timestamp)
                n3870 = To Double Precision Float(number=w4627) -> (double precision float=→"START 2":dbl)
                n3871 = local write "FLAG"(100.0 ("FLAG")) -> ()
              }
            }
          }
        }
        n3872 = disable-structure shown="Disabled" {
          disable-tunnel: w4605 -> [w4614 _]
          disable-tunnel: [w4613 _] -> w4604
          frame Disabled {
            n3873 = local read "Json St Flg"() -> (w4612:bool)
            n3874 = case shown="True" w4612 {
              tunnel: w4614 -> [w4615 w4617]
              tunnel: [w4615 w4616] -> w4613
              frame False {
              }
              frame True {
                n3875 = Increment(x=w4617) -> (x+1=w4616:dbl)
                "T cycle" <- w4616
                n3876 = local write "Json St Flg"(FALSE ("Json St Flg")) -> ()
              }
            }
          }
          frame Enabled {
          }
        }
        n3877 = local read "Quit"() -> (w4599:bool)
      }
    }
    frame Enabled {
    }
  }
  n3878 = stacked-sequence {
    tunnel: [w4997] -> w38
    frame #0 {
      w4997 = FALSE ("Upload \nConfirmed")
      n3879 = local write "Upload \nConfirmed"(w4997) -> ()
      n3880 = local write "St Str"("") -> ()
    }
  }
  n3881 = disable-structure shown="Disabled" {
    disable-tunnel: w38 -> [w4998 _]
    frame Disabled {
      n3882 = case shown="True" {
        selector: _ -> [_ _]
        tunnel: w4998 -> [_ w4999]
        frame False {
        }
        frame True {
          n3883 = while {
            tunnel: [w5005] -> _
            tunnel: w4999 -> [_]
            i -> [w5005]
            stop <- w5000 stop-if-true
            n3884 = local read "Json End Flg"() -> (w5004:bool)
            n3885 = Wait (ms)(milliseconds to wait=u32 20 ("Refresh Rate (ms)")) -> ()  [unwired: 1 out]
            n3886 = local read "refresh flag"() -> (w5001:bool)
            n3887 = local read "RUN"() -> (w5002:bool)
            n3888 = And(x=w5002, y=w5001) -> (x .and. y?=w5003:bool)
            n3889 = Or(x=w5003, y=w5004) -> (x .or. y?=w5006:bool)
            "AR Led" <- w5006
            n3890 = case shown="True" w5006 {
              frame False {
              }
              frame True {
                w5023 = "\",\""
                n3891 = local read "UUID"() -> (w5021:string)
                n3892 = local write "refresh flag"(FALSE ("refresh flag")) -> ()
                n3893 = local read "time"() -> (w5010:dbl)
                n3894 = Multiply(x=w5010, y=60.0) -> (x*y=w5009:dbl)
                n3895 = Concatenate Strings("UUID\" : \"", w5021, "\"}") -> (w5024:string)
                n3896 = Number To Fractional String(number=w5009, width (-)=i16 10, precision (6)=i16 4) -> (F-format string=w5038:string)  [unwired: 1 in]
                n3897 = Concatenate Strings("{", "\"Time\":\"", w5038, w5023) -> (w5033:string)
                n3898 = stacked-sequence {
                  tunnel: w5023 -> [w5086 w5094 w5101 w5109 w5117 w5126 w5133]
                  tunnel: [w5087 _ _ _ _ _ _] -> w5037
                  tunnel: [_ w5095 _ _ _ _ _] -> w5036
                  tunnel: [_ _ w5102 _ _ _ _] -> w5035
                  tunnel: [_ _ _ w5111 _ _ _] -> w5034
                  tunnel: w5024 -> [_ _ _ _ _ _ w5144]
                  tunnel: [_ _ _ _ _ _ w5143] -> w5020
                  tunnel: [_ _ _ _ _ w5123 _] -> w5019
                  tunnel: [_ _ _ _ w5116 _ _] -> w5018
                  frame #0 {
                    n3899 = local read "NORMAL LOAD"() -> (w5085:dbl)
                    n3900 = Number To Fractional String(number=w5085, width (-)=i16 10, precision (6)=i16 4) -> (F-format string=w5088:string)  [unwired: 1 in]
                    n3901 = Concatenate Strings("NormalLoad\":\"", w5088, w5086) -> (w5087:string)
                  }
                  frame #1 {
                    n3902 = local read "Temp"() -> (w5093:dbl)
                    n3903 = Number To Fractional String(number=w5093, width (-)=i16 10, precision (6)=i16 4) -> (F-format string=w5096:string)  [unwired: 1 in]
                    n3904 = Concatenate Strings("Temperature\":\"", w5096, w5094) -> (w5095:string)
                  }
                  frame #2 {
                    n3905 = local read "cof"() -> (w5099:dbl)
                    n3906 = Number To Fractional String(number=w5099, width (-)=i16 10, precision (6)=i16 4) -> (F-format string=w5103:string)  [unwired: 1 in]
                    n3907 = Concatenate Strings("FrictionalForce\":\"", w5103, w5101) -> (w5102:string)
                  }
                  frame #3 {
                    n3908 = local read "Set Hz"() -> (w5107:dbl)
                    n3909 = Multiply(x=w5107, y=60.0) -> (x*y=w5106:dbl)
                    n3910 = Number To Fractional String(number=w5106, width (-)=i16 10, precision (6)=i16 4) -> (F-format string=w5112:string)  [unwired: 1 in]
                    n3911 = Concatenate Strings("Speed\":\"", w5112, w5109) -> (w5111:string)
                  }
                  frame #4 {
                    n3912 = local read item#-1() -> (w5115)
                    n3913 = Number To Fractional String(number=w5115, width (-)=i16 10, precision (6)=i16 4) -> (F-format string=w5119:string)  [unwired: 1 in]
                    n3914 = Concatenate Strings("LinearDeformation\":\"", w5119, w5117) -> (w5116:string)
                  }
                  frame #5 {
                    n3915 = local read "AIR TEMP"() -> (w5122:dbl)
                    n3916 = local read "Json St Flg"() -> (w5124:bool)
                    n3917 = local read "Json End Flg"() -> (w5125:bool)
                    n3918 = Number To Fractional String(number=w5122, width (-)=i16 10, precision (6)=i16 4) -> (F-format string=w5128:string)  [unwired: 1 in]
                    n3919 = Concatenate Strings("Vibration\":\"", w5128, w5126) -> (w5123:string)
                    n3920 = And(x=w5124, y=w5125) -> ()  [unwired: 1 out]
                  }
                  frame #6 {
                    n3921 = local read "Json End Flg"() -> (w5132:bool)
                    n3922 = Get Date/Time In Seconds() -> (seconds since 1Jan1904=w5140:timestamp)
                    n3923 = local read "Json St Flg"() -> (w5131:bool)
                    n3924 = To Double Precision Float(number=w5140) -> (double precision float=w5139:dbl)
                    n3925 = Subtract(x=w5139, y=2082844800.0) -> (x-y=w5137:dbl)
                    n3926 = Number To Fractional String(number=w5137, width (-)=i16 12, precision (6)=i16 0) -> (F-format string=w5134:string)  [unwired: 1 in]
                    n3927 = case shown="True" w5132 {
                      tunnel: ["" w5147] -> w5141
                      tunnel: w5134 -> [_ w5148]
                      tunnel: w5133 -> [_ w5146]
                      frame False {
                      }
                      frame True {
                        n3928 = local write "Json End Flg"(FALSE ("Json St Flg")) -> ()
                        n3929 = Concatenate Strings("End\": \"", w5148, w5146) -> (w5147:string)
                      }
                    }
                    n3930 = case shown="True" w5131 {
                      tunnel: [w5151 w5154] -> w5142
                      tunnel: w5134 -> [_ w5155]
                      tunnel: w5133 -> [_ w5152]
                      frame False {
                        n3931 = local read "St Str"() -> (w5151:string)
                      }
                      frame True {
                        n3932 = Concatenate Strings("Start\":\"", w5155, w5152) -> (w5154:string)
                        "St Str" <- w5154
                        n3933 = local write "Json St Flg"(FALSE ("Json St Flg")) -> ()
                      }
                    }
                    n3934 = Concatenate Strings(w5142, w5141, w5144) -> (w5143:string)
                  }
                }
                n3935 = local read "FILE"() -> (w5012:string)
                n3936 = Concatenate Strings("\",\"OperatorID\":\"" ("string"), "Operator ID") -> (w5015:string)
                n3937 = Concatenate Strings("\",\"DatasetTitle\":\"" ("string"), w5012) -> (w5014:string)
                n3938 = Concatenate Strings("\",\"SerialNumber\":\"" ("string"), "Serial No") -> (w5044:string)
                n3939 = Concatenate Strings("\",\"ModelNumber\":\"" ("string"), "Model No") -> (w5043:string)
                n3940 = Concatenate Strings(w5044, w5043) -> (w5026:string)
                n3941 = Concatenate Strings("{\"SecretKey\":\"", "Secret Key", w5026, w5015, w5014, "\",\"Samples\":[") -> (w5031:string)
                n3942 = Concatenate Strings(w5033, w5037, w5036, w5035, w5034, w5018, w5019, w5020) -> (w5032:string)
                n3943 = Concatenate Strings(w5031, w5032, "]}") -> (w5030:string)
                n3944 = stacked-sequence {
                  tunnel: w5030 -> [w5059 _ _]
                  tunnel: [_ _ w5076] -> _
                  frame #0 {
                    (unwired) FALSE ("convert eol (F)")
                    w5061 = enum16{"start", "end", "current"}."start" ("pos mode (0:2)")
                    n3945 = Path To String(path="Path") -> (string=w5067:string)
                    n3946 = Concatenate Strings(w5067, "\\", "Data File Name") -> (w5069:string)
                    n3947 = local write "standard output"(" ") -> ()
                    n3948 = String To Path(string=w5069) -> (path=w5058:path)
                    n3949 = call <vilib>:"Open_Create_Replace File.vi"("advisory dialog? (display:T)"=FALSE, "function (open:0)"=T31."create or replace", "file path"=w5058) -> ("error out"=w5072:errorcluster, "refnum"=w5071:refnum<file>)  [unwired: 5 in, 2 out]
                    n3950 = Set File Position(refnum=w5071, from (0:start)=w5061, error in=w5072) -> (refnum out=w5052:refnum<file>, error out=w5051:errorcluster)  [unwired: 1 in]
                    n3951 = Write to Binary File(file (use dialog)=w5052, data=" ", error in=w5051, 5:FALSE ("prepend array or string size? (T)")) -> (refnum out=w5062:refnum<file>, error out=w5063:errorcluster)  [unwired: 2 in, 1 out]
                    n3952 = Set File Position(offset (in bytes) (0)=w5061, refnum=w5062, error in=w5063) -> (refnum out=w5055:refnum<file>, error out=w5054:errorcluster)  [unwired: 1 in]
                    n3953 = Write to Binary File(file (use dialog)=w5055, data=w5059, error in=w5054, 5:FALSE ("prepend array or string size? (T)")) -> (error out=w5057:errorcluster)  [unwired: 2 in, 2 out]
                    n3954 = flat-sequence {
                      tunnel: w5058 -> [w5074]
                      tunnel: w5057 -> [_]
                      frame #0 {
                        n3955 = call <vilib>:"Read Characters From File.vi"("file path (dialog if empty)"=w5074) -> ("character string"=→"JSON string":string)  [unwired: 5 in, 3 out]
                      }
                    }
                    "SinglePoint" <- w5059
                  }
                  frame #1 {
                  }
                  frame #2 {
                    (unwired) "\"Stored\": true" ("string")
                    n3956 = call <vilib>:"System Exec.vi"("run minimized? (F)"=TRUE, "wait until completion? (T)"=TRUE, "working directory"=path "C:/LAB-IQ-NXT", "command line"="C:\\LAB-IQ-NXT\\JPost.bat") -> ("standard error"=→"Respose From Server":string, "standard output"=w5079:string)  [unwired: 4 in, 2 out]
                    "standard output" <- w5079
                    n3957 = Match Pattern(string=w5079, regular expression="JSON Check String") -> (match substring=w5077:string, offset past match=w5076:i32)  [unwired: 1 in, 2 out]
                    n3958 = Equal?(x=w5077, y="JSON Check String") -> (x = y?=→"Upload \nConfirmed":bool)
                  }
                }
              }
            }
            n3959 = local read "Quit"() -> (w5000:bool)
          }
        }
      }
    }
    frame Enabled {
    }
  }
  n3960 = disable-structure shown="Disabled" {
    disable-tunnel: _ -> [w5162 _]
    frame Disabled {
      n3961 = while {
        shift-right: [w5170] -> w5158
        shift-left: _ -> [w5171]
        shift-right: [w5168] -> w5159
        shift-left: errorcluster {"status"=TRUE, "code"=0, "source"="Init"} ("error out") -> [w5169]
        shift-right: [w5166] -> _
        shift-left: "" -> [w5167]
        tunnel: [w5164] -> _
        tunnel: w5162 -> [_]
        i -> [w5164]
        stop <- w5163 stop-if-true
        n3962 = flat-sequence {
          tunnel: [w5172] -> w5165
          frame #0 {
            n3963 = Wait (ms)(milliseconds to wait=10.0 ("Delay")) -> (millisecond timer value=w5172:u32)
          }
        }
        n3964 = case shown="No Error" w5169 {
          selector: w5169 -> [w5202 w5321]
          tunnel: [w5185 w5323] -> w5170
          tunnel: [w5184 w5322] -> w5168
          tunnel: w5171 -> [w5203 w5315]
          tunnel: w5167 -> [w5183 w5314]
          tunnel: [w5182 w5314] -> w5166
          tunnel: w5165 -> [_ _]
          frame No Error {
            n3965 = Concatenate Strings("\r", "\n") -> (w5194:string)  [unwired: 1 in]
            n3966 = case shown="True" w5195 {
              tunnel: w5203 -> [w5227 w5234]
              tunnel: w5202 -> [w5226 w5233]
              tunnel: [w5227 w5232] -> w5201
              tunnel: [w5226 w5231] -> w5181
              tunnel: w5194 -> [_ w5230]
              frame False {
              }
              frame True {
                n3967 = VISA Write(VISA resource name=w5234, write buffer=w5230, error in (no error)=w5233) -> (VISA resource name out=w5232:refnum<visa-resource-name>, error out=w5231:errorcluster)  [unwired: 1 out]
                n3968 = local write "Read String"("") -> ()
                n3969 = local write item#-1(FALSE) -> ()
              }
            }
            n3970 = property class="Instr"(reference=w5201, error in=w5181) -> (reference out=w5200:refnum<visa-resource-name>, error out=w5199:errorcluster, "Serial Settings:Number of Bytes at Serial Port"=w5198:u32)
            n3971 = Greater?(x=w5198, y=u32 100) -> (0:w5196:bool)
            n3972 = case shown="True" w5196 {
              tunnel: w5200 -> [w5237 w5261]
              tunnel: w5199 -> [w5236 w5260]
              tunnel: w5198 -> [_ w5259]
              tunnel: [w5237 w5258] -> w5187
              tunnel: [w5236 w5257] -> w5186
              tunnel: w5183 -> [w5235 w5256]
              tunnel: [w5235 ""] -> w5182
              frame False {
              }
              frame True {
                w5246 = u32 6 ("y")
                # "Page 84 of \nmanual"
                n3973 = VISA Read(VISA resource name=w5261, byte count=w5259, error in (no error)=w5260) -> (VISA resource name out=w5258:refnum<visa-resource-name>, read buffer=w5254:string, error out=w5257:errorcluster)  [unwired: 1 out]
                n3974 = while {
                  tunnel: w5254 -> [w5310]
                  tunnel: [w5306] -> w5248 mode=indexing
                  tunnel: [w5300] -> w5252 mode=indexing
                  tunnel: [w5298] -> _
                  i -> [w5298]
                  stop <- w5303 stop-if-true
                  n3975 = String Subset(string=w5310, offset (0)=w5298) -> (substring=w5305:string)  [unwired: 1 in]
                  n3976 = String To Byte Array(string=w5305) -> (unsigned byte array=w5309:u8[])
                  n3977 = String Length(string=w5305) -> (length=w5304:i32)
                  n3978 = Index Array(array=w5309) -> (element=w5308:u8)  [unwired: 1 in]
                  n3979 = Equal To 0?(x=w5304) -> (x = 0?=w5303:bool)
                  n3980 = Number To Boolean Array(number=w5308) -> (Boolean array=w5302:bool[])
                  n3981 = Reverse 1D Array(array=w5302) -> (reversed array=w5301:bool[])
                  n3982 = And(x=w5302, y=bool[] [FALSE, FALSE, FALSE, FALSE, FALSE, FALSE, TRUE, TRUE] ("Boolean array")) -> (x .and. y?=w5306:bool[])
                  n3983 = And(x=w5301, y=bool[] [FALSE, FALSE, TRUE, TRUE, TRUE, TRUE, TRUE, TRUE] ("Boolean array")) -> (x .and. y?=w5300:bool[])
                }
                n3984 = Concatenate Strings(w5256, w5254) -> (→"Read String":string)
                n3985 = while {
                  tunnel: w5248 -> [w5297] mode=indexing
                  tunnel: [w5293] -> w5251
                  i -> [w5293]
                  stop <- w5294 stop-if-true
                  n3986 = Search 1D Array(1D array=w5297, element=TRUE) -> (index of element=w5295:i32)  [unwired: 1 in]
                  n3987 = Less Than 0?(x=w5295) -> (x < 0?=w5294:bool)
                }
                n3988 = Delete From Array(array=w5252, length=w5251, index (row)=0) -> (array with subset deleted=w5247:bool[][])  [unwired: 1 in, 1 out]
                n3989 = Array Size(array=w5247) -> (size(s)=w5249:i32[])
                n3990 = Index Array(array=w5249) -> (element=w5241:i32)  [unwired: 1 in]
                n3991 = Greater?(x=w5241, y=w5246) -> (0:w5244:bool)
                n3992 = Subtract(x=w5241, y=w5246) -> (x-y=w5245:u32)
                n3993 = Select(t=w5245, s=w5244, f=u32 0) -> (s? t:f=w5242:u32)
                n3994 = while {
                  tunnel: w5247 -> [w5280]
                  tunnel: [w5282] -> w5240 mode=indexing
                  tunnel: w5242 -> [w5264]
                  i -> [w5281]
                  stop <- w5279 stop-if-true
                  w5271 = 6 ("index")
                  w5270 = 2 ("length")
                  # "Page 65 of \nmanual"
                  n3995 = Multiply(x=u32 3 ("y"), y=w5281) -> (x*y=w5278:u32)
                  n3996 = Divide(x=u32 102 ("y"), y=u32 65520) -> (x/y=w5288:dbl)
                  n3997 = Greater Or Equal?(x=w5278, y=w5264) -> (x >= y?=w5279:bool)
                  n3998 = Index Array(array=w5280, index (row) #1=w5278) -> (element #1=w5276:bool[], element #2=w5275:bool[], element #3=w5274:bool[])  [unwired: 5 in]
                  n3999 = Reverse 1D Array(array=w5276) -> (reversed array=w5269:bool[])
                  n4000 = Reverse 1D Array(array=w5275) -> (reversed array=w5273:bool[])
                  n4001 = Reverse 1D Array(array=w5274) -> (reversed array=w5272:bool[])
                  n4002 = Delete From Array(array=w5269, length=w5270, index=w5271) -> (array with subset deleted=w5265:bool[])  [unwired: 1 out]
                  n4003 = Delete From Array(array=w5273, length=w5270, index=w5271) -> (array with subset deleted=w5266:bool[])  [unwired: 1 out]
                  n4004 = Delete From Array(array=w5272, length=w5270, index=w5271) -> (array with subset deleted=w5267:bool[])  [unwired: 1 out]
                  n4005 = Insert Into Array(array=bool[] [] ("Boolean array"), new element #1=w5265, new element #2=w5266, new element #3=w5267) -> (w5268:bool[])  [unwired: 1 in]
                  n4006 = Boolean Array To Number(Boolean array=w5268) -> (number=w5277:u32)
                  n4007 = Multiply(x=w5288, y=w5277) -> (x*y=w5287:dbl)
                  n4008 = Decrement(x=w5287) -> (x-1=w5286:dbl)
                  n4009 = Divide(x=w5286, y=u32 100) -> (x/y=w5284:dbl)
                  n4010 = Multiply(x=w5284, y=u32 10) -> (x*y=w5282:dbl)
                }
                n4011 = Delete From Array(array=w5240) -> (array with subset deleted=w5239:dbl[])  [unwired: 2 in, 1 out]
                "Waveform Graph 5" <- w5239
                "Waveform Chart 3" <- w5239
                n4012 = call-poly <vilib>:"Mean.vi"("X"=w5239) -> ("mean"=w5238:dbl)  [unwired: 1 out]
                n4013 = case shown="True" {
                  selector: _ -> [_ _]
                  tunnel: w5238 -> [_ w5263]
                  frame False {
                  }
                  frame True {
                    n4014 = local write item#-1(FALSE ("Zero 4")) -> ()
                    "z_measure" <- w5263
                  }
                }
              }
            }
            n4015 = local read item#-1() -> (w5178)
            n4016 = local read item#-1() -> (w5177)
            n4017 = local read item#-1() -> (w5179)
            n4018 = local read item#-1() -> (w5176)
            n4019 = case shown="True" w5174 {
              tunnel: w5178 -> [_ w5206]
              tunnel: w5179 -> [_ w5205]
              frame False {
              }
              frame True {
                n4020 = Build Array(w5206, w5205) -> (w5204:void[])
                n4021 = local read item#-1() -> (w5209)
                n4022 = Build Array (concatenate)(w5209, w5204) -> (w5207:void[])
                n4023 = local write item#-1(w5207) -> ()
                n4024 = local write item#-1(FALSE ("Boolean 8")) -> ()
              }
            }
            n4025 = call "Build XY Graph"("Enable"=w5176, "Reset"=w5177, "Y Input"=w5179, "X Input"=w5178) -> ("XY Graph"=w5175:cluster{"Y":dbl[], "Y":dbl[]}[])  [unwired: 6 in, 1 out]
            n4026 = case shown="True" {
              selector: _ -> [_ _]
              frame False {
              }
              frame True {
                n4027 = local read item#-1() -> (w5210)
                n4028 = Index Array(array=w5210, index (col) #1=0 ("disabled index (col)"), index (col) #2=1 ("index (col)")) -> (element #1=w5212, element #2=w5211)  [unwired: 2 in]
                n4029 = call <vilib>:"Linear Fit.vi"("Y"=w5212, "X"=w5211) -> ()  [unwired: 9 in, 5 out]
                n4030 = local write item#-1(FALSE ("Boolean 9")) -> ()
              }
            }
            n4031 = case shown="True" {
              selector: _ -> [_ _]
              frame False {
              }
              frame True {
                n4032 = local write item#-1(dbl[][] [] ("Captured Values")) -> ()
                n4033 = local write item#-1(FALSE ("Boolean 7")) -> ()
              }
            }
            n4034 = Concatenate Strings("\r", "\n") -> (w5189:string, w5188:string)
            n4035 = case shown="True" w5180 {
              tunnel: w5187 -> [w5219 w5225]
              tunnel: w5186 -> [w5218 w5224]
              tunnel: [w5219 w5223] -> w5185
              tunnel: [w5218 w5222] -> w5184
